vi "getEmuPerPixel.vi"(8 "error in (no error)":errorcluster) -> (0 "error out":errorcluster, 3 "EMU_PER_PIXEL":i32)   [LabVIEW 2017]
uses:
  C:/Users/Neo/Desktop/Dev_Tools_BR/LabVIEW_NPOI/lib/NPOI 2.1.1/NPOI.OOXML.dll
  lib/NPOI 2.1.1/NPOI.OOXML.dll
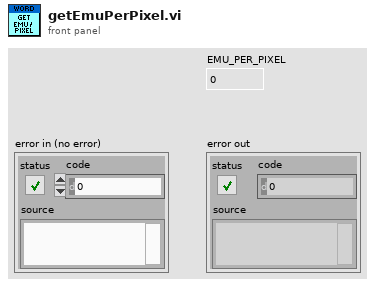
[diagram p1: front panel]
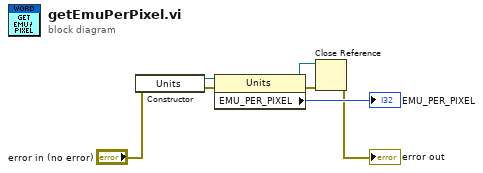
[diagram p0: block diagram]
diagram:
  n1 = constructor class="Units"(error in="error in (no error)") -> (reference out=w7:refnum<k24>, error out=w6:errorcluster)  [unwired: 2 in, 1 out]
  n2 = property class="Units"(reference=w7, error in=w6) -> (reference out=w5:refnum<k24>, error out=w4:errorcluster, "EMU_PER_PIXEL"=→"EMU_PER_PIXEL":i32)
  n3 = Close Reference(reference=w5, error in (no error)=w4) -> (error out=→"error out":errorcluster)
